vi "RVC 6-link serial robot with tool 2014.vi"() -> ()   [LabVIEW 2014]
uses:
  <vilib>/robotics/Kinematics/Robot/Robot Pose.ctl
  <vilib>/Analysis/baseanly.llb/Real A x B.vi
  <vilib>/Analysis/_algsub.llb/Vector Norm.vi
  <vilib>/Analysis/_algsub.llb/Real Vector Norm.vi
  <vilib>/Analysis/baseanly.llb/Outer Product.vi
  <vilib>/Analysis/baseanly.llb/Real Outer Product.vi
  <vilib>/robotics/Kinematics/Create Lie Group Matrix.vi
  <vilib>/robotics/Kinematics/Analytical/Initialize Generic Serial Arm.vi
  <vilib>/Analysis/7linalg.llb/Create Special Matrix.vi
  <vilib>/Analysis/7linalg.llb/Create Special Real Matrix.vi
  <vilib>/Analysis/Matrix/Numeric/Multiply/Multiply.vi
  <vilib>/Analysis/Matrix/Numeric/Multiply/Multiply - RM,R.vi
  <vilib>/Analysis/Matrix/Numeric/Multiply/Multiply - R,RM.vi
  <vilib>/Analysis/Matrix/Numeric/Add/Add.vi
  <vilib>/Analysis/Matrix/Numeric/Add/Add - RM,RM.vi
  <vilib>/robotics/Kinematics/Analytical/NI_Robotics_AnalyticKinematics.lvlib
  <vilib>/robotics/Kinematics/Link/Joint Type.ctl
  <vilib>/robotics/Kinematics/Link/NI_Robotics_Link.lvclass
  <vilib>/robotics/Kinematics/Robot/NI_Robotics_Serial Robot Arm.lvclass
  <vilib>/robotics/Kinematics/NI_Kinematics.lvlib
  <vilib>/Analysis/NI_AALBase.lvlib
panel:
  in  "Ring":u16(ring) items=["Origin", "Above", "Up-side down"]
  in  "End-Effector Offcenter":bool
  out "transformation":picture
  in  "Pose":u16(ring) items=["qz", "qr", "qs", "qn"]
  in  "stop":bool
  out "3D Picture":refnum<vi>(3d-picture)
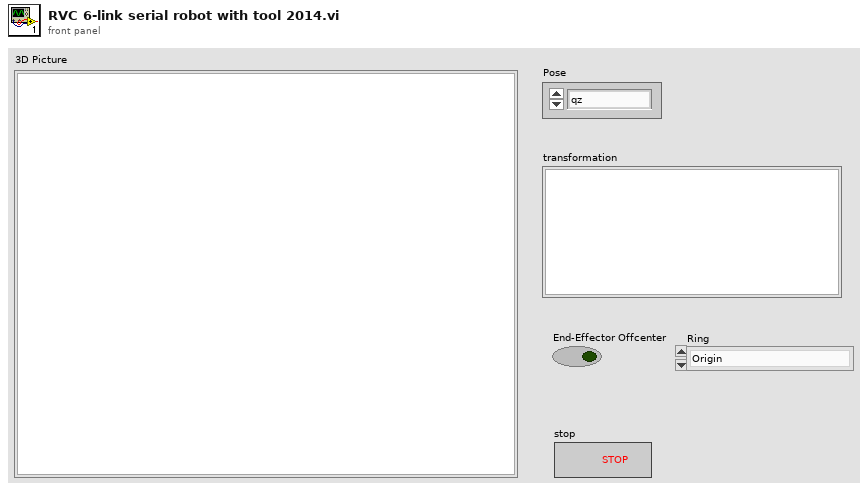
[diagram p1: front panel]
types:
  T1 = typedef "NI_Robotics_Serial Robot Arm.lvclass/Robot Pose.ctl" = cluster{"name":string, "description":string, "joint positions":dbl[]}
  T2 = typedef "NI_Robotics_Link.lvclass/Joint Type.ctl" = enum16{"Revolute", "Prismatic"}
  T3 = cluster{"Twist Angle":dbl, "Length":dbl, "Rotation Angle":dbl, "Offset Distance":dbl, "Joint Type":T2, "Joint Coordinate Offset":dbl}[]
  T4 = typedef "DH Kinematic Parameters.ctl" = cluster{"twist angle":dbl, "length":dbl, "rotation angle":dbl, "offset distance":dbl, "joint type":T2, "joint coordinate offset":dbl}
  T5 = typedef "NI_Matrix.lvlib/RealMatrix.ctl" = dbl[][]
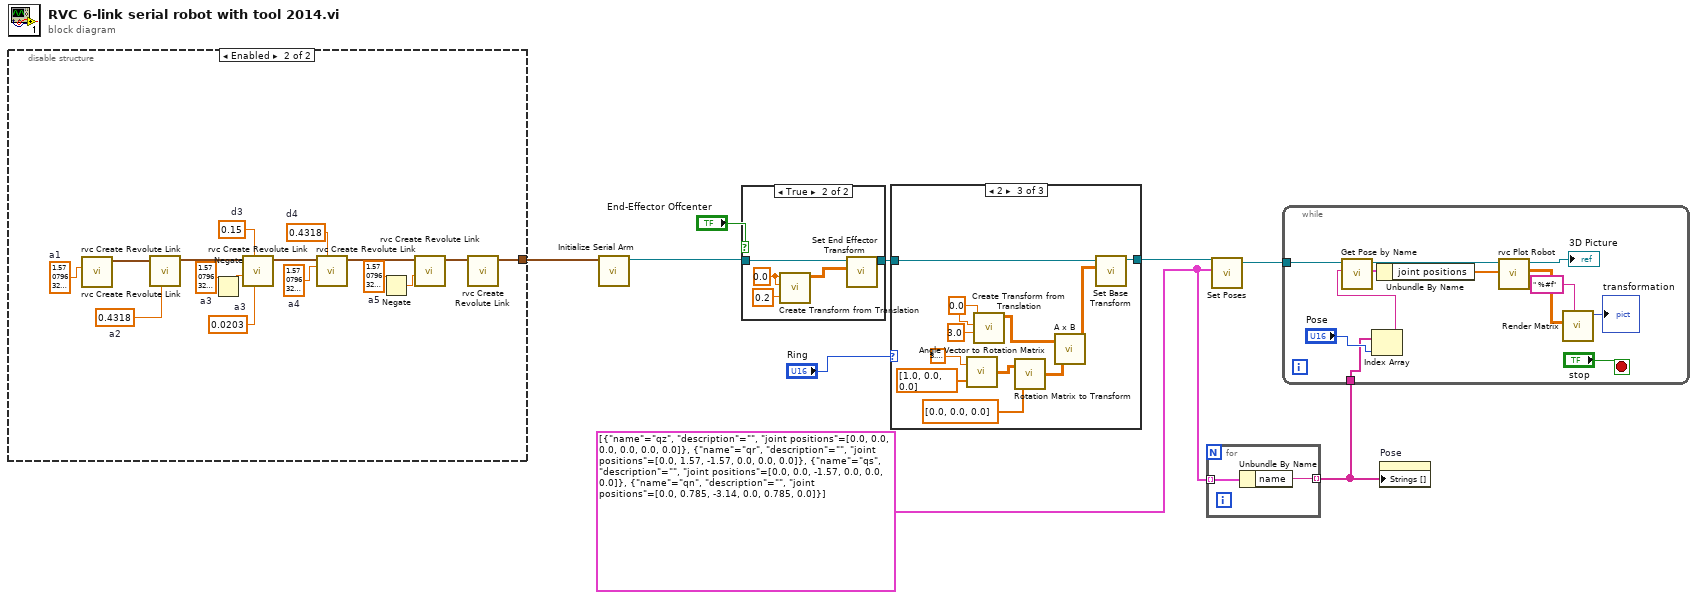
[diagram p0: block diagram]
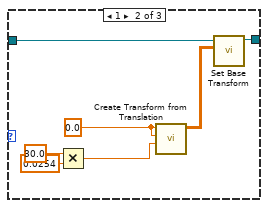
[diagram p3: hidden frame]
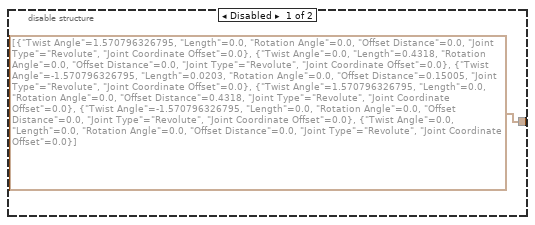
[diagram p5: hidden frame]
diagram:
  w7 = T1[] [{"name"="qz", "description"="", "joint positions"=[0.0, 0.0, 0.0, 0.0, 0.0, 0.0]}, {"name"="qr", "description"="", "joint positions"=[0.0, 1.57, -1.57, 0.0, 0.0, 0.0]}, {"name"="qs", "description"="", "joint positions"=[0.0, 0.0, -1.57, 0.0, 0.0, 0.0]}, {"name"="qn", "description"="", "joint positions"=[0.0, 0.785, -3.14, 0.0, 0.785, 0.0]}] ("serial arm poses")
  n1 = disable-structure shown="Enabled" {
    disable-tunnel: [T3 [{"Twist Angle"=1.570796326795, "Length"=0.0, "Rotation Angle"=0.0, "Offset Distance"=0.0, "Joint Type"=enum."Revolute", "Joint Coordinate Offset"=0.0}, {"Twist Angle"=0.0, "Length"=0.4318, "Rotation Angle"=0.0, "Offset Distance"=0.0, "Joint Type"=enum."Revolute", "Joint Coordinate Offset"=0.0}, {"Twist Angle"=-1.570796326795, "Length"=0.0203, "Rotation Angle"=0.0, "Offset Distance"=0.15005, "Joint Type"=enum."Revolute", "Joint Coordinate Offset"=0.0}, {"Twist Angle"=1.570796326795, "Length"=0.0, "Rotation Angle"=0.0, "Offset Distance"=0.4318, "Joint Type"=enum."Revolute", "Joint Coordinate Offset"=0.0}, {"Twist Angle"=-1.570796326795, "Length"=0.0, "Rotation Angle"=0.0, "Offset Distance"=0.0, "Joint Type"=enum."Revolute", "Joint Coordinate Offset"=0.0}, {"Twist Angle"=0.0, "Length"=0.0, "Rotation Angle"=0.0, "Offset Distance"=0.0, "Joint Type"=enum."Revolute", "Joint Coordinate Offset"=0.0}] w25] -> w9
    frame Disabled {
    }
    frame Enabled {
      w12 = 1.5707963267948966  # a5
      w13 = 0.4318  # d4
      w14 = 1.5707963267948966  # a4
      w16 = 1.5707963267948966  # a3
      w17 = 0.15  # d3
      w18 = 0.0203  # a3
      w22 = 0.4318  # a2
      w24 = 1.5707963267948966  # a1
      n2 = call "rvc Create Revolute Link.vi"("twist angle (alpha)"=w24) -> ("Array"=w23:T4[])  [unwired: 10 in]
      n3 = call "rvc Create Revolute Link.vi"("length (a)"=w22, "Array 2"=w23) -> ("Array"=w21:T4[])  [unwired: 9 in]
      n4 = Negate(x=w16) -> (-x=w15:dbl)
      n5 = call "rvc Create Revolute Link.vi"("length (a)"=w18, "offset distance (d)"=w17, "twist angle (alpha)"=w15, "Array 2"=w21) -> ("Array"=w20:T4[])  [unwired: 7 in]
      n6 = call "rvc Create Revolute Link.vi"("offset distance (d)"=w13, "twist angle (alpha)"=w14, "Array 2"=w20) -> ("Array"=w19:T4[])  [unwired: 8 in]
      n7 = Negate(x=w12) -> (-x=w11:dbl)
      n8 = call "rvc Create Revolute Link.vi"("twist angle (alpha)"=w11, "Array 2"=w19) -> ("Array"=w26:T4[])  [unwired: 9 in]
      n9 = call "rvc Create Revolute Link.vi"("Array 2"=w26) -> ("Array"=w25:T4[])  [unwired: 10 in]
    }
  }
  n10 = call-poly <vilib>:"Initialize Serial Arm.vi"("kinematic parameters"=w9) -> ("serial arm out"=w5:refnum<class "NI_Robotics_Serial Robot Arm.lvclass">)  [unwired: 9 in, 1 out]
  n11 = case shown="True" "End-Effector Offcenter" {
    tunnel: w5 -> [w27 w32]
    tunnel: [w27 w28] -> w4
    frame False {
    }
    frame True {
      w29 = 0.0 ("x")
      n12 = call <vilib>:"Create Transform from Translation.vi"("z"=0.2, "y"=w29, "x"=w29) -> ("transform"=w31:T5)  [unwired: 8 in]
      n13 = call <vilib>:"Set End Effector Transform.vi"("end effector transform"=w31, "serial arm in"=w32) -> ("serial arm out"=w28:refnum<class "NI_Robotics_Serial Robot Arm.lvclass">)  [unwired: 8 in, 1 out]
    }
  }
  n14 = case shown="2" "Ring" {
    tunnel: w4 -> [w33 w40 w51]
    tunnel: [w33 w39 w50] -> w3
    frame 0, Default {
    }
    frame 1 {
      w37 = 0.0 ("x")
      n15 = Multiply(x=30.0, y=0.0254) -> (x*y=w36:dbl)
      n16 = call <vilib>:"Create Transform from Translation.vi"("z"=w36, "y"=w37, "x"=w37) -> ("transform"=w38:T5)  [unwired: 8 in]
      n17 = call <vilib>:"Set Base Transform.vi"("base transform"=w38, "serial arm in"=w40) -> ("serial arm out"=w39:refnum<class "NI_Robotics_Serial Robot Arm.lvclass">)  [unwired: 8 in, 1 out]
    }
    frame 2 {
      w47 = 0.0 ("z")
      n18 = call <vilib>:"Angle Vector to Rotation Matrix.vi"("vector"=dbl[] [1.0, 0.0, 0.0], "angle"=3.141592653589793) -> ("rotation matrix"=w43:T5)
      n19 = call <vilib>:"Create Transform from Translation.vi"("z"=3.0, "y"=w47, "x"=w47) -> ("transform"=w48:T5)  [unwired: 8 in]
      n20 = call <vilib>:"Rotation Matrix to Transform.vi"("translation vector"=dbl[] [0.0, 0.0, 0.0], "rotation matrix"=w43) -> ("transform"=w42:T5)
      n21 = call-poly <vilib>:"A x B.vi"("B"=w42, "A"=w48) -> ("A x B"=w49:T5)  [unwired: 1 out]
      n22 = call <vilib>:"Set Base Transform.vi"("base transform"=w49, "serial arm in"=w51) -> ("serial arm out"=w50:refnum<class "NI_Robotics_Serial Robot Arm.lvclass">)  [unwired: 8 in, 1 out]
    }
  }
  n23 = for {
    tunnel: w7 -> [w53] mode=indexing
    tunnel: [w52] -> w6 mode=indexing
    n24 = Unbundle By Name(w53) -> ("name"=w52:string)
  }
  n25 = call <vilib>:"Set Poses.vi"("serial arm poses"=w7, "serial arm in"=w3) -> ("serial arm out"=w8:refnum<class "NI_Robotics_Serial Robot Arm.lvclass">)  [unwired: 8 in, 1 out]
  n26 = while {
    tunnel: w8 -> [w62]
    tunnel: w6 -> [w58]
    stop <- "stop" stop-if-true
    n27 = Index Array(array=w58, index="Pose") -> (element=w57:string)
    n28 = call <vilib>:"Get Pose by Name.vi"("name"=w57, "serial arm in"=w62) -> ("serial arm pose"=w64:T1, "serial arm out"=w61:refnum<class "NI_Robotics_Serial Robot Arm.lvclass">)  [unwired: 7 in, 1 out]
    n29 = Unbundle By Name(w64) -> ("joint positions"=w63:dbl[])
    n30 = call "rvc Plot Robot.vi"("joint positions"=w63, "NI_Robotics_Serial Robot Arm in"=w61) -> ("forward kinematics"=w56:T5, "Scene Object Out"=→"3D Picture":refnum<vi>)  [unwired: 8 in]
    n31 = call "Render Matrix.vi"("format string"=" %#f", "A"=w56) -> ("picture out"=→"transformation":picture)  [unwired: 9 in]
  }
  n32 = property on="Pose" class="Ring (strict)"("Strings []"=w6) -> ()  [unwired: 2 in, 2 out]
